vi "Czysc buf Wfm.vi"(11 "Wfm Bufor in":waveform(dbl)[](array[waveform])) -> (3 "Array":waveform(dbl)[](array[waveform]))   [LabVIEW 2014]
doc: "Czyœci bufor danych"
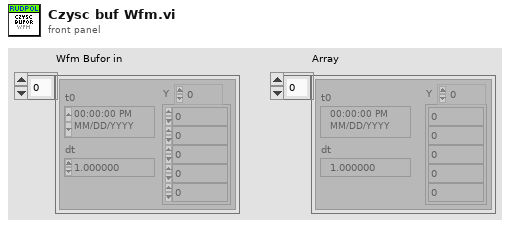
[diagram p1: front panel]
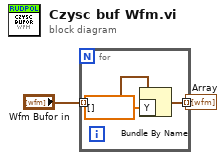
[diagram p0: block diagram]
diagram:
  n1 = for {
    tunnel: "Wfm Bufor in" -> [w5] mode=indexing
    tunnel: [w4] -> w2 mode=indexing
    n2 = Bundle By Name(cluster=w5, "Y"=dbl[] []) -> (w4:waveform(dbl))
  }
  "Array" <- w2
